vi "Array.vi"() -> ()   [LabVIEW 2019]
panel:
  in  "StringArray":string[](array[string])
  in  "IntArray":u8[](array[numeric])
  in  "FloatArray":dbl[](array[numeric])
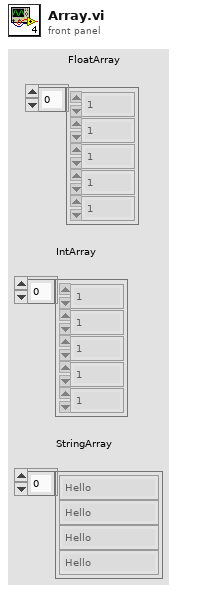
[diagram p1: front panel]
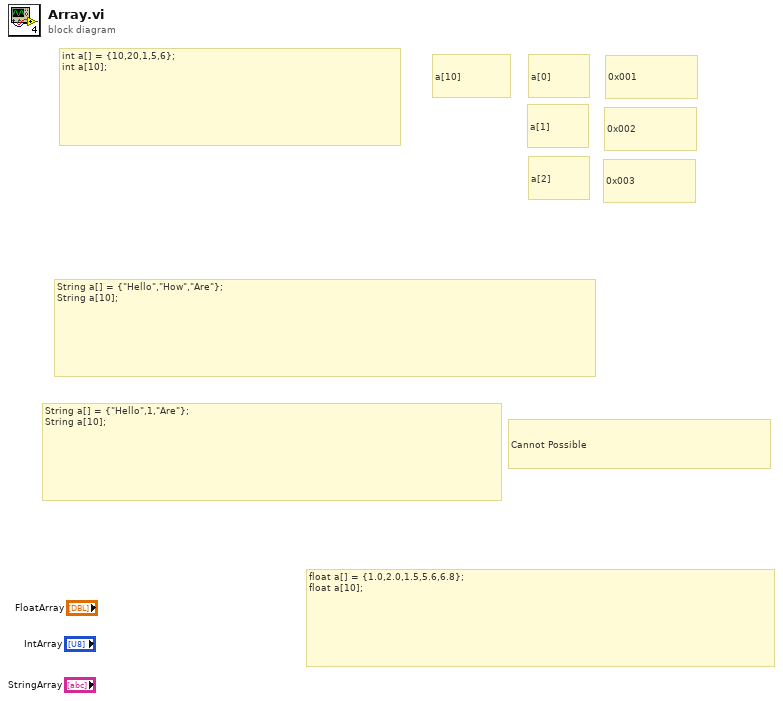
[diagram p0: block diagram]
diagram:
  # "Cannot Possible"
  # "String a[] = {\"Hello\",1,\"Are\"};\nString a[10];"
  # "String a[] = {\"Hello\",\"How\",\"Are\"};\nString a[10];"
  # "float a[] = {1.0,2.0,1.5,5.6,6.8};\nfloat a[10];"
  # "0x003"
  # "a[2]"
  # "0x002"
  # "a[1]"
  # "0x001"
  # "a[0]"
  # "a[10]"
  # "int a[] = {10,20,1,5,6};\nint a[10];"
